vi "Read Digital Input Port.vi"(8 "error in (no error)":errorcluster, 10 "Input Port Number (0)":i32, 11 "VISA resource name":refnum<visa-resource-name>) -> (0 "error out":errorcluster, 2 "Port Status":bool, 3 "VISA resource name out":refnum<visa-resource-name>)   [LabVIEW 2017, in "HH PLI Series.lvlib"]
doc: "Reads digital input ports."
uses:
  HH PLI Series.lvlib
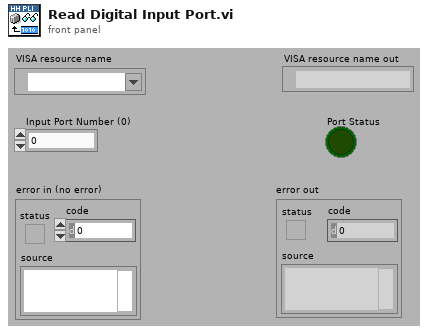
[diagram p1: front panel]
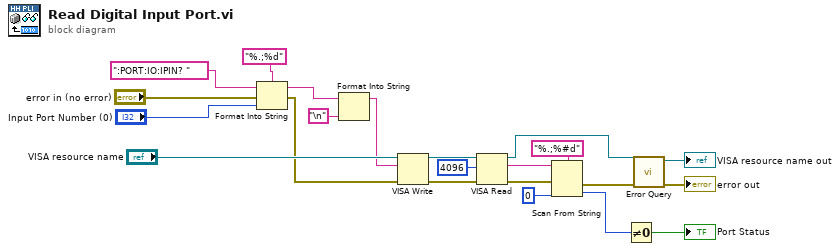
[diagram p0: block diagram]
diagram:
  n1 = Format Into String(format string="%.;%d", initial string=":PORT:IO:IPIN? " ("command"), error in="error in (no error)", "Input Port Number (0)") -> (resulting string=w3:string, error out=w20:errorcluster)
  n2 = Format Into String(initial string=w3, "\n") -> (resulting string=w1:string)  [unwired: 2 in, 1 out]
  n3 = VISA Write(VISA resource name="VISA resource name", write buffer=w1, error in (no error)=w20) -> (VISA resource name out=w18:refnum<visa-resource-name>, error out=w17:errorcluster)  [unwired: 1 out]
  n4 = VISA Read(VISA resource name=w18, byte count=u32 4096, error in (no error)=w17) -> (VISA resource name out=w5:refnum<visa-resource-name>, read buffer=w15:string, error out=w13:errorcluster)  [unwired: 1 out]
  n5 = Scan From String(format string="%.;%#d", input string=w15, error in=w13, default 1=0 ("default value 1")) -> (error out=w8:errorcluster, output 1=w10:i32)  [unwired: 1 in, 2 out]
  n6 = Not Equal To 0?(x=w10) -> (x != 0?=→"Port Status":bool)
  n7 = call "Error Query.vi"("error in (no error)"=w8, "VISA resource name"=w5) -> ("error out"=→"error out":errorcluster, "VISA resource name out"=→"VISA resource name out":refnum<visa-resource-name>)  [unwired: 6 in, 2 out]
